vi "abre_aplicacao_adq.vi"() -> ()   [LabVIEW 2019]
panel:
  in  "editar":bool
  in  "Sair":bool
  in  "Abrir Configuracao":bool
  # "ADQUIRI"
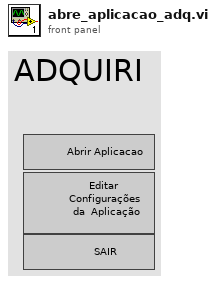
[diagram p1: front panel]
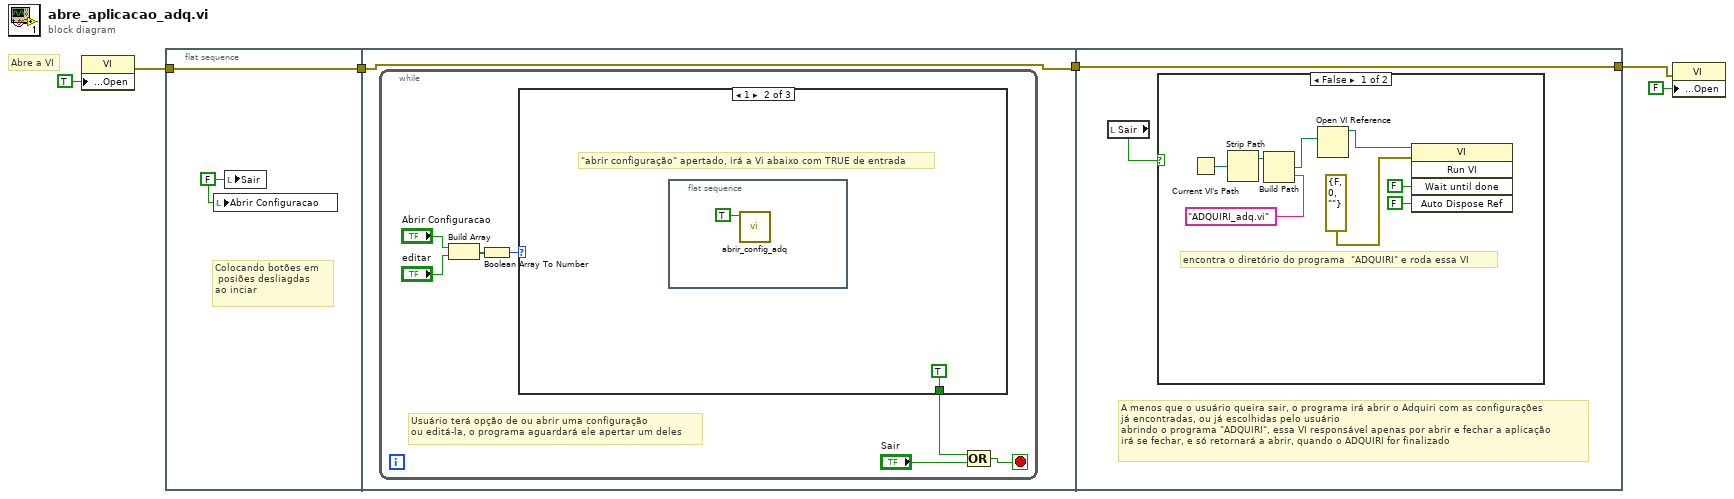
[diagram p0: block diagram]
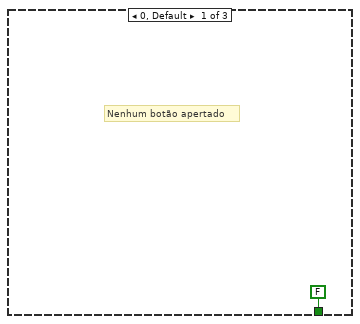
[diagram p2: hidden frame]
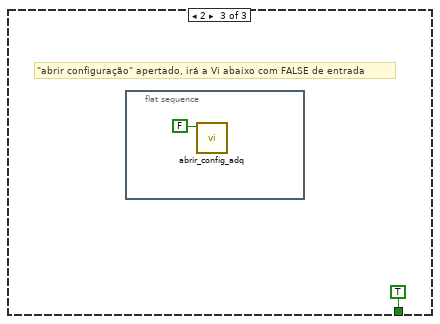
[diagram p3: hidden frame]
diagram:
  # "Abre a VI"
  n1 = property class="VI"("Front Panel.Open"=TRUE ("Front Panel Window:Open")) -> (error out=w3:errorcluster)  [unwired: 2 in, 1 out]
  n2 = flat-sequence {
    tunnel: [w8] -> w4
    tunnel: w3 -> [w8]
    tunnel: [w9] -> w6
    tunnel: w4 -> [w9]
    tunnel: w6 -> [w22]
    tunnel: [w22] -> w1
    frame #0 {
      w7 = FALSE ("Sair")
      # "Colocando botões em\n posiões desliagdas \nao inciar"
      n3 = local write "Abrir Configuracao"(w7) -> ()
      n4 = local write "Sair"(w7) -> ()
    }
    frame #1 {
      n5 = while {
        stop <- w16 stop-if-true
        # "Usuário terá opção de ou abrir uma configuração\nou editá-la, o programa aguardará ele apertar um deles"
        n6 = Build Array("Abrir Configuracao", "editar") -> (w10:bool[])
        n7 = Boolean Array To Number(Boolean array=w10) -> (number=w11:u32)
        n8 = case shown="1" w11 {
          tunnel: [FALSE ("SALVAR 2") TRUE ("file or folder exists?") TRUE ("file or folder exists?")] -> w14
          frame 0, Default {
            # "Nenhum botão apertado"
          }
          frame 1 {
            # "\"abrir configuração\" apertado, irá a Vi abaixo com TRUE de entrada"
            n9 = flat-sequence {
              frame #0 {
                n10 = call "abrir_config_adq.vi"("ABRIR"=TRUE) -> ()  [unwired: 11 in]
              }
            }
          }
          frame 2 {
            # "\"abrir configuração\" apertado, irá a Vi abaixo com FALSE de entrada"
            n11 = flat-sequence {
              frame #0 {
                n12 = call "abrir_config_adq.vi"("ABRIR"=FALSE) -> ()  [unwired: 11 in]
              }
            }
          }
        }
        n13 = Compound Arithmetic op=OR(w14, "Sair") -> (w16:bool)
      }
    }
    frame #2 {
      # "A menos que o usuário queira sair, o programa irá abrir o Adquiri com as configurações\njá encontradas, ou já escolhidas pelo usuário\nabrindo o programa \"ADQUIRI\", essa VI responsável apenas por abrir e fechar a aplicação\nirá se fechar, e só retornará a abrir, quando o ADQUIRI for finalizado"
      n14 = local read "Sair"() -> (w23:bool)
      n15 = case shown="False" w23 {
        frame False {
          # "encontra o diretório do programa  \"ADQUIRI\" e roda essa VI"
          n16 = Current VI's Path() -> (path=w28:path)
          n17 = Strip Path(path=w28) -> (stripped path=w27:path)  [unwired: 1 out]
          n18 = Build Path(base path=w27, name or relative path="ADQUIRI_adq.vi") -> (appended path=w25:path)
          n19 = Open VI Reference(vi path=w25) -> (vi reference=w24:refnum<vi>)  [unwired: 5 in, 1 out]
          n20 = invoke class="VI" method="Run VI"(reference=w24, error in=errorcluster {"status"=FALSE, "code"=0, "source"=""} ("error in (no error)"), "Wait until done"=FALSE ("Wait Until Done"), "Auto Dispose Ref"=FALSE ("Auto Dispose Reference")) -> ()  [unwired: 1 in, 5 out]
        }
        frame True {
        }
      }
    }
  }
  n21 = property class="VI"(error in=w1, "Front Panel.Open"=FALSE ("Front Panel Window:Open")) -> ()  [unwired: 1 in, 2 out]
